vi "Teleop.vi"(8 "error in (no error)":errorcluster, 9 "Joystick Data":T2, 10 "Robot Data In":T1, 11 "Panzer in":refnum<class "Panzer.lvclass">) -> (0 "error out":errorcluster, 2 "Robot Data Out":T1, 3 "Panzer out":refnum<class "Panzer.lvclass">)   [LabVIEW 2019, in "Robot.lvlib" / "Panzer.lvclass"]
uses:
  Panzer.lvclass
  Joysticks/Controls/JoystickData.ctl
  TypeDefs/RobotObjects.ctl
  Robot.lvclass
  Drive/Tank Drive/Tank Drive.lvclass
  Pnematics control/Pneumatics.lvclass
  Vision/Vision.lvclass
  Joysticks/Joysticks.lvclass
  Elevator/Elevator.lvclass
  Hatch/Hatch.lvclass
  Cargo/Cargo.lvclass
  DriveOld/Drive.lvclass
  Control Panel/Control Panel.lvclass
  Climber/Climber.lvclass
  Turret/Turret.lvclass
  PowerCellHandler/Power Cell Handler.lvclass
  Pnematics control/Solenoids/Solenoids.lvclass
panel:
  out "Boolean":bool
  in  "Air Cool":dbl=95.0 format="%#_13g"
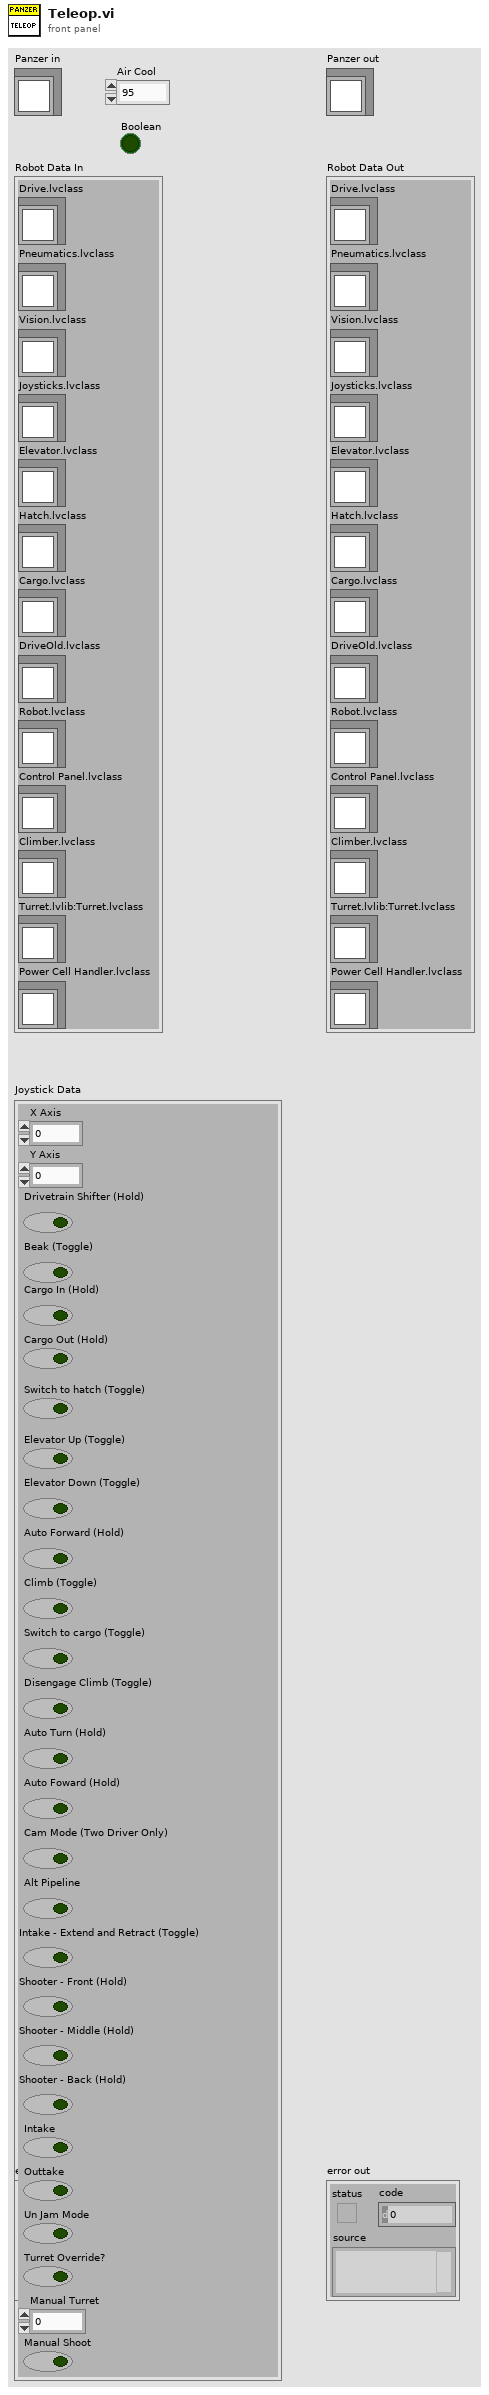
[diagram p1: front panel]
types:
  T1 = typedef "RobotObjects.ctl" = cluster{"Drive.lvclass":refnum<class "Tank Drive.lvclass">, "Pneumatics.lvclass":refnum<class "Pneumatics.lvclass">, "Vision.lvclass":refnum<class "Vision.lvclass">, "Joysticks.lvclass":refnum<class "Joysticks.lvclass">, "Elevator.lvclass":refnum<class "Elevator.lvclass">, "Hatch.lvclass":refnum<class "Hatch.lvclass">, "Cargo.lvclass":refnum<class "Cargo.lvclass">, "DriveOld.lvclass":refnum<class "Drive.lvclass">, "Robot.lvclass":refnum<class "Robot.lvclass">, "Control Panel.lvclass":refnum<class "Control Panel.lvclass">, "Climber.lvclass":refnum<class "Climber.lvclass">, "Turret.lvlib:Turret.lvclass":refnum<class "Turret.lvclass">, "Power Cell Handler.lvclass":refnum<class "Power Cell Handler.lvclass">}
  T2 = typedef "Joysticks.lvlib/Joysticks.lvclass/JoystickData.ctl" = cluster{"X Axis ":dbl, "Y Axis":dbl, "Drivetrain Shifter (Hold)":bool, "Beak (Toggle)":bool, "Cargo In (Hold)":bool, "Cargo Out (Hold)":bool, "Switch to hatch (Toggle)":bool, "Elevator Up (Toggle)":bool, "Elevator Down (Toggle)":bool, "Auto Forward (Hold)":bool, "Climb (Toggle)":bool, "Switch to cargo (Toggle)":bool, "Disengage Climb (Toggle)":bool, "Auto Turn (Hold)":bool, "Auto Foward (Hold)":bool, "Cam Mode (Two Driver Only)":bool, "Alt Pipeline":bool, "Intake - Extend and Retract (Toggle)":bool, "Shooter - Front (Hold)":bool, "Shooter - Middle (Hold)":bool, "Shooter - Back (Hold)":bool, "Intake":bool, "Outtake":bool, "Un Jam Mode":bool, "Turret Override?":bool, "Manual Turret":dbl, "Manual Shoot":bool}
  T3 = typedef "Power Cell Handler.lvlib/Power Cell Handler.lvclass/Shooting Position.ctl" = enum16{"Rest", "Front", "Middle", "Back"}
  T4 = typedef "Turret.lvlib/Turret.lvclass/Turret control states.ctl" = enum16{"Position", "Offset", "IMU"}
  T5 = typedef "Drive.lvlib/Tank Drive.lvclass/Drive Train Temperatures.ctl" = cluster{"Left Lead Temperature (C)":dbl, "Right Lead Temperature (C)":dbl, "Left Follows Temperatures (C)":dbl[], "Right Follows Temperatures (C)":dbl[]}
  T6 = typedef "Pneumatics control.lvlib/Pneumatics.lvclass/Solenoids.ctl" = cluster{"Air Cooler":refnum<class "Solenoids.lvclass">, "ArmLock":refnum<class "Solenoids.lvclass">, "HatchArm":refnum<class "Solenoids.lvclass">, "HatchGrabber":refnum<class "Solenoids.lvclass">, "CPDeploy":refnum<class "Solenoids.lvclass">, "Power Cells Intake":refnum<class "Solenoids.lvclass">}
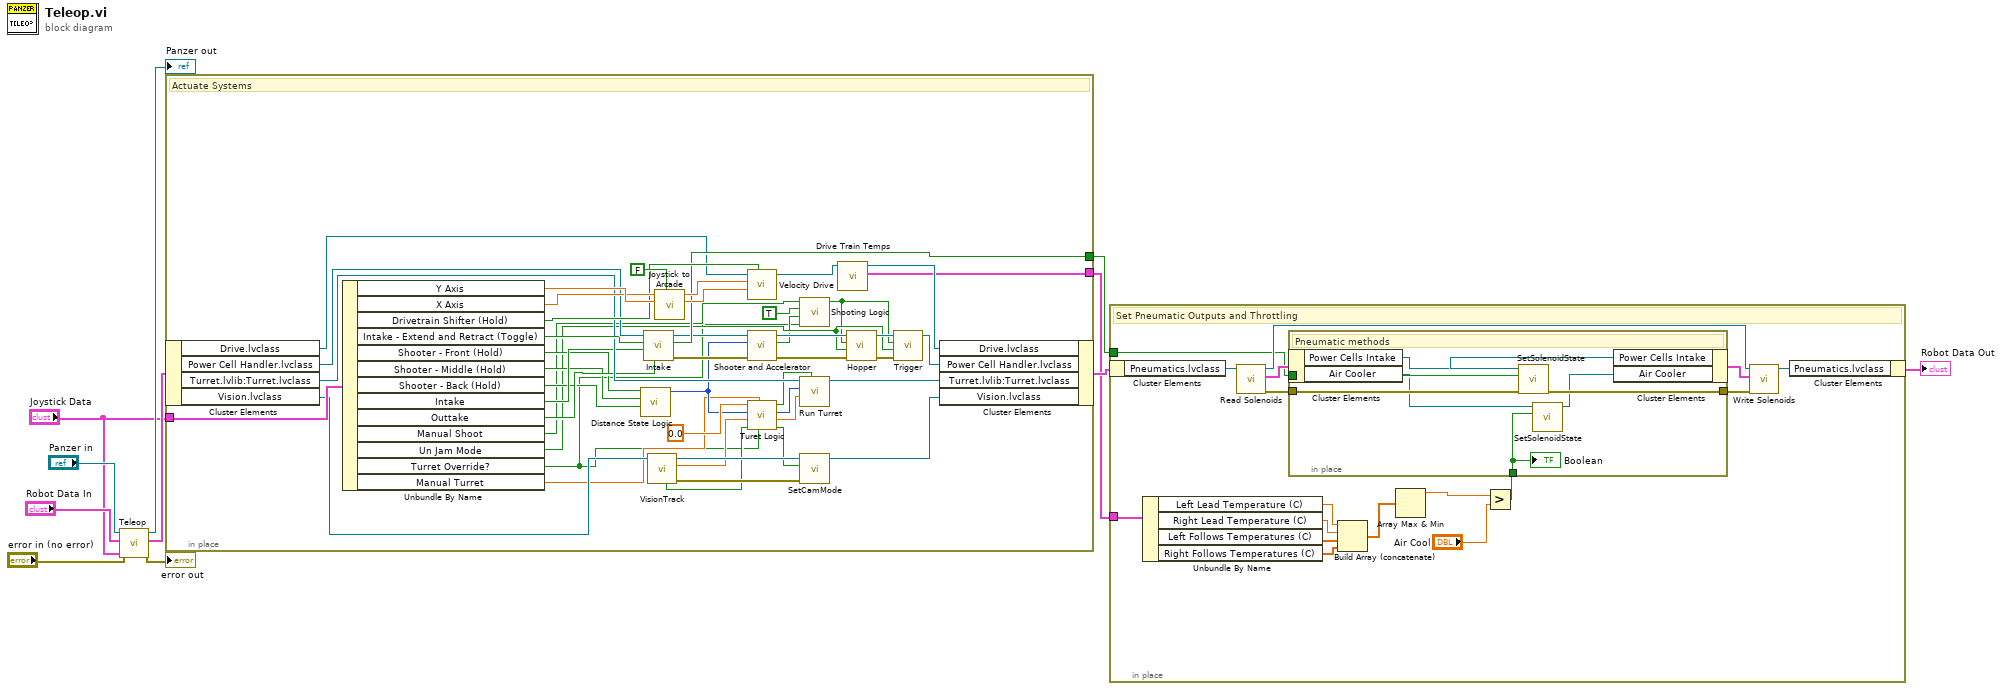
[diagram p0: block diagram]
diagram:
  n1 = call-parent "Teleop.vi"("error in (no error)"="error in (no error)", "Joystick Data"="Joystick Data", "Robot Data In"="Robot Data In", "Robot in"="Panzer in") -> ("error out"=→"error out":errorcluster, "Robot Data Out"=w6:T1, "Robot out"=→"Panzer out":refnum<class "Panzer.lvclass">)  [unwired: 5 in]
  n2 = in-place {
    in-place-border: "Joystick Data" -> [w52]
    in-place-border: [w49] -> w2
    in-place-border: [w12] -> w1
    # "Actuate Systems"
    n3 = in-place-cluster #1(w6) -> ("Drive.lvclass"=w15:refnum<class "Tank Drive.lvclass">, "Power Cell Handler.lvclass"=w51:refnum<class "Power Cell Handler.lvclass">, "Turret.lvlib:Turret.lvclass"=w48:refnum<class "Turret.lvclass">, "Vision.lvclass"=w40:refnum<class "Vision.lvclass">)
    n4 = Unbundle By Name(w52) -> ("Y Axis"=w55:dbl, "X Axis"=w54:dbl, "Drivetrain Shifter (Hold)"=w53:bool, "Intake - Extend and Retract (Toggle)"=w50:bool, "Shooter - Front (Hold)"=w27:bool, "Shooter - Middle (Hold)"=w26:bool, "Shooter - Back (Hold)"=w25:bool, "Intake"=w31:bool, "Outtake"=w30:bool, "Manual Shoot"=w24:bool, "Un Jam Mode"=w20:bool, "Turret Override?"=w16:bool, "Manual Turret"=w19:dbl)
    n5 = call "Distance State Logic.vi"("Back"=w25, "Mid"=w26, "Front"=w27) -> ("Shooting State"=w23:T3)  [unwired: 8 in]
    n6 = call "Intake.vi"("intake reversed?"=w30, "Intake Running?"=w31, "Intake Out?"=w50, "Power Cell Handler in"=w51) -> ("error out"=w36:errorcluster, "Deploy Intake"=w49:bool, "Power Cell Handler out"=w37:refnum<class "Power Cell Handler.lvclass">)  [unwired: 5 in]
    n7 = call "VisionTrack.vi"("Vision in"=w40) -> ("error out"=w42:errorcluster, "HorizontalOffset(degrees)"=w29:dbl, "Vision out"=w43:refnum<class "Vision.lvclass">, "Target?"=w22:bool)  [unwired: 5 in, 2 out]
    n8 = call "Joystick to Arcade.vi"("Negate Right input (true)"=FALSE, "Forward"=w55, "Right"=w54) -> ("Right Wheel"=w57:dbl, "Left Wheel"=w58:dbl)  [unwired: 7 in]
    n9 = call-dynamic "Velocity Drive.vi"("High Gear?"=w53, "Right Speed"=w57, "Left Speed"=w58, "Tank Drive in"=w15) -> ("Tank Drive out"=w14:refnum<class "Tank Drive.lvclass">)  [unwired: 6 in, 1 out]
    n10 = call "Shooter and Accelerator.vi"("error in (no error)"=w36, "Shooting Position"=w23, "Power Cell Handler in"=w37) -> ("error out"=w35:errorcluster, "Ready to fire"=w18:bool, "Power Cell Handler out"=w33:refnum<class "Power Cell Handler.lvclass">)  [unwired: 6 in]
    n11 = call "Turet Logic.vi"("Turret Override?"=w16, "Manual Turret"=w19, "Vision Target?"=w22, "Vision Xoffset"=w29, "Shooting Position"=w23, "Driver Xoffset"=0.0) -> ("Activate vision"=w41:bool, "Turret Offset(degrees)"=w45:dbl, "Turret mode"=w46:T4, "Scan Mode"=w44:bool)  [unwired: 2 in]
    n12 = call "Shooting Logic.vi"("Shoot Override?"=w16, "Ready to Fire?"=w18, "In Range?"=TRUE, "is gunner ready to shoot?"=w24) -> ("Shooting"=w17:bool)  [unwired: 7 in]
    n13 = call "Run Turret.vi"("Search?"=w44, "Input(deg)"=w45, "Control mode"=w46, "Turret in"=w48) -> ("Turret out"=w47:refnum<class "Turret.lvclass">)  [unwired: 5 in, 2 out]
    n14 = call "SetCamMode.vi"("Vision.lvlib:Vision.lvclass"=w43, "Vision Processing?"=w41, "error in (no error)"=w42) -> ("Vision.lvlib:Vision.lvclass"=w39:refnum<class "Vision.lvclass">)  [unwired: 6 in, 1 out]
    n15 = call-dynamic "Drive Train Temps.vi"("Tank Drive in"=w14) -> ("Drive Train Temperatures"=w12:T5, "Tank Drive out"=w13:refnum<class "Tank Drive.lvclass">)  [unwired: 8 in, 1 out]
    n16 = call "Hopper.vi"("error in (no error)"=w35, "Un Jam Mode"=w20, "Shooting"=w17, "Power Cell Handler in"=w33) -> ("error out"=w34:errorcluster, "Power Cell Handler out"=w32:refnum<class "Power Cell Handler.lvclass">)  [unwired: 6 in]
    n17 = call "Trigger.vi"("error in (no error)"=w34, "Un Jam Mode"=w20, "Shooting"=w17, "Power Cell Handler in"=w32) -> ("Power Cell Handler out"=w38:refnum<class "Power Cell Handler.lvclass">)  [unwired: 6 in, 1 out]
    n18 = in-place-cluster #1("Drive.lvclass"=w13, "Power Cell Handler.lvclass"=w38, "Turret.lvlib:Turret.lvclass"=w47, "Vision.lvclass"=w39) -> (w9:T1)
  }
  n19 = in-place {
    in-place-border: w2 -> [w68]
    in-place-border: w1 -> [w67]
    # "Set Pneumatic Outputs and Throttling"
    n20 = in-place-cluster #2(w9) -> ("Pneumatics.lvclass"=w71:refnum<class "Pneumatics.lvclass">)
    n21 = Unbundle By Name(w67) -> ("Left Lead Temperature (C)"=w64:dbl, "Right Lead Temperature (C)"=w63:dbl, "Left Follows Temperatures (C)"=w62:dbl[], "Right Follows Temperatures (C)"=w61:dbl[])
    n22 = call-dynamic "Read Solenoids.vi"("Pneumatics in"=w71) -> ("error out"=w73:errorcluster, "Solenoids"=w74:T6, "Pneumatics out"=w75:refnum<class "Pneumatics.lvclass">)  [unwired: 8 in]
    n23 = Build Array (concatenate)(w64, w63, w62, w61) -> (w60:dbl[])
    n24 = Array Max & Min(array=w60) -> (max value=w65:dbl)  [unwired: 3 out]
    n25 = Greater?(x=w65, y="Air Cool") -> (0:w59:bool)
    n26 = in-place {
      in-place-border: w73 -> [w82]
      in-place-border: [w80] -> w69
      in-place-border: w68 -> [w79]
      in-place-border: w59 -> [w77]
      # "Pneumatic methods"
      n27 = in-place-cluster #3(w74) -> ("Power Cells Intake"=w81:refnum<class "Solenoids.lvclass">, "Air Cooler"=w78:refnum<class "Solenoids.lvclass">)
      n28 = call-dynamic "SetSolenoidState.vi"("error in (no error)"=w82, "Solenoid On?"=w79, "Solenoids in"=w81) -> ("error out"=w80:errorcluster, "Solenoids out"=w83:refnum<class "Solenoids.lvclass">)  [unwired: 7 in]
      n29 = call-dynamic "SetSolenoidState.vi"("Solenoid On?"=w77, "Solenoids in"=w78) -> ("Solenoids out"=w76:refnum<class "Solenoids.lvclass">)  [unwired: 8 in, 1 out]
      n30 = in-place-cluster #3("Power Cells Intake"=w83, "Air Cooler"=w76) -> (w72:T6)
      "Boolean" <- w77
    }
    n31 = call-dynamic "Write Solenoids.vi"("error in (no error)"=w69, "Solenoids"=w72, "Pneumatics in"=w75) -> ("Pneumatics out"=w70:refnum<class "Pneumatics.lvclass">)  [unwired: 7 in, 1 out]
    n32 = in-place-cluster #2("Pneumatics.lvclass"=w70) -> (→"Robot Data Out":T1)
  }
